vi "Profil Y.vi"(8 "error in (no error)":errorcluster caption="entrée d'erreur (pas d'erreur)", 10 "Image in":T1(plugin-control), 11 "Acq Cam Basler en entrée":refnum<class "Acq Cam Basler.lvclass">) -> (0 "error out":errorcluster caption="sortie d'erreur", 2 "Image out":T1(plugin-control), 3 "Acq Cam Basler en sortie":refnum<class "Acq Cam Basler.lvclass">)   [LabVIEW 2023, in "Acq Cam Basler.lvclass"]
uses:
  Acq Cam Basler.lvclass
  Acq Cam Basler.lvclass/Acq Cam Basler.ctl
  <vilib>/vision/NI_Vision_Development_Module.lvlib
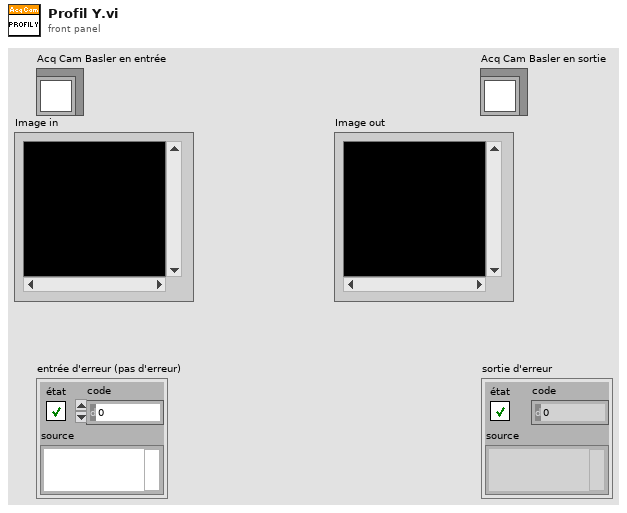
[diagram p1: front panel]
types:
  T1 = typedef "IMAQ Image.ctl" = refnum<image>
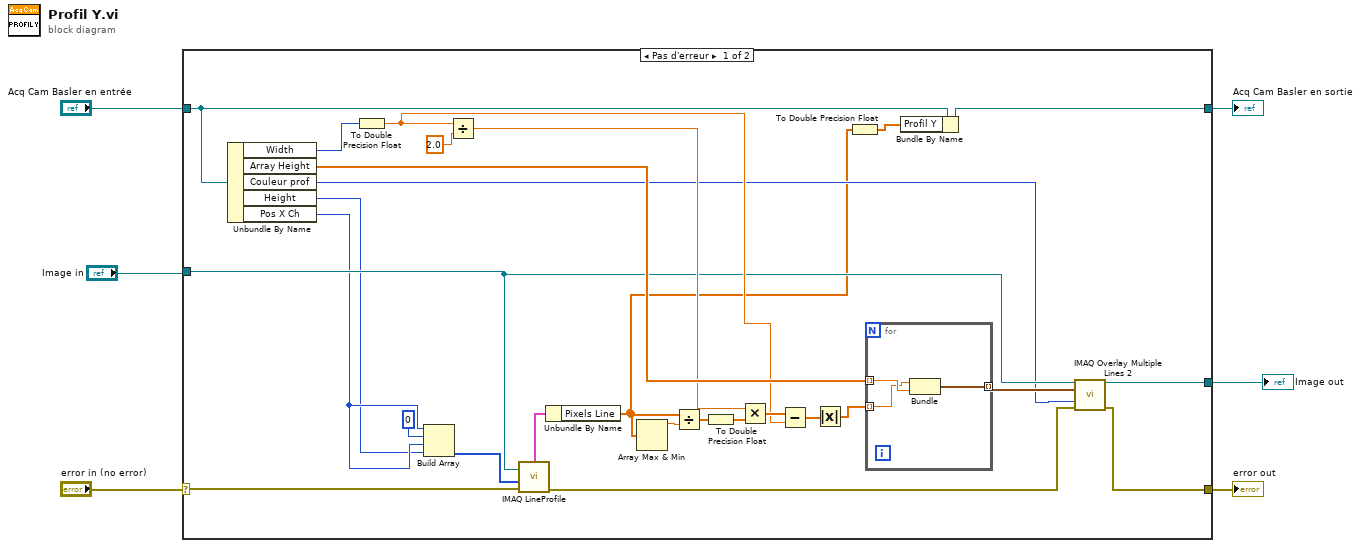
[diagram p0: block diagram]
diagram:
  n1 = case shown="Pas d'erreur" "error in (no error)" {
    selector: "error in (no error)" -> [w31 w39]
    tunnel: [w15 w39] -> w5
    tunnel: [w9 w38] -> w3
    tunnel: "Acq Cam Basler en entrée" -> [w33 w38]
    tunnel: "Image in" -> [w17 w37]
    tunnel: [w14 w37] -> w1
    frame No Error {
      n2 = Unbundle By Name(w33) -> ("Width"=w30:u32, "Array Height"=w27:dbl[], "Couleur prof"=w10:u32, "Height"=w11:u32, "Pos X Ch"=w12:u32)
      n3 = To Double Precision Float(number=w30) -> (double precision float=w20:dbl)
      n4 = Build Array(w12, u32 0 ("élément"), w12, w11) -> (w32:u32[])
      n5 = Divide(x=w20, y=2.0) -> (x/y=w22:dbl)
      n6 = call "IMAQ LineProfile"("error in (no error)"=w31, "Line Coordinates"=w32, "Image"=w17) -> ("error out"=w16:errorcluster, "Line Graph"=w28:cluster{"x0":sgl, "dx":sgl, "Pixels Line":sgl[]})  [unwired: 2 in, 2 out]
      n7 = Unbundle By Name(w28) -> ("Pixels Line"=w8:sgl[])
      n8 = Array Max & Min(array=w8) -> (max value=w26:sgl)  [unwired: 3 out]
      n9 = Divide(x=w8, y=w26) -> (x/y=w25:sgl[])
      n10 = To Double Precision Float(number=w25) -> (double precision float=w24:dbl[])
      n11 = Multiply(x=w22, y=w24) -> (x*y=w23:dbl[])
      n12 = Subtract(x=w23, y=w20) -> (x-y=w21:dbl[])
      n13 = Absolute Value(x=w21) -> (abs(x)=w19:dbl[])
      n14 = To Double Precision Float(number=w8) -> (double precision float=w7:dbl[])
      n15 = for {
        tunnel: w27 -> [w35] mode=indexing
        tunnel: w19 -> [w34] mode=indexing
        tunnel: [w36] -> w18 mode=indexing
        n16 = Bundle(w34, "Numérique"=w35) -> (w36:cluster{dbl, "Numérique":dbl})  [unwired: 1 in]
      }
      n17 = Bundle By Name(cluster=w33, "Profil Y"=w7) -> (w9:refnum<class "Acq Cam Basler.lvclass">)
      n18 = call "IMAQ Overlay Multiple Lines 2"("Image"=w17, "Line End Points"=w18, "Color"=w10, "error in (no error)"=w16) -> ("Image Out"=w14:T1, "error out"=w15:errorcluster)  [unwired: 10 in]
    }
    frame Error {
    }
  }
  "error out" <- w5
  "Acq Cam Basler en sortie" <- w3
  "Image out" <- w1
